vi "Configure Rate.vi"(7 "auto timeout (s)":enum16{"1s", "5s", "10s", "20s"}(ring), 8 "error in":errorcluster, 9 "time (ms)":T1(ring), 10 "option":enum16{"TIME", "AUTO"}(ring), 11 "VISA resource name":refnum<visa-resource-name>) -> (0 "error out":errorcluster, 3 "VISA resource out":refnum<visa-resource-name>)   [LabVIEW 2018, in "Suita SPAW7000.lvlib"]
uses:
  <instrlib>/Suita SPAW7000/Suita SPAW7000.lvlib
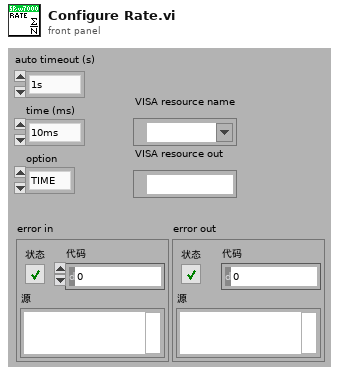
[diagram p1: front panel]
types:
  T1 = enum16{"10ms", "50ms", "100ms", "250ms", "500ms"}
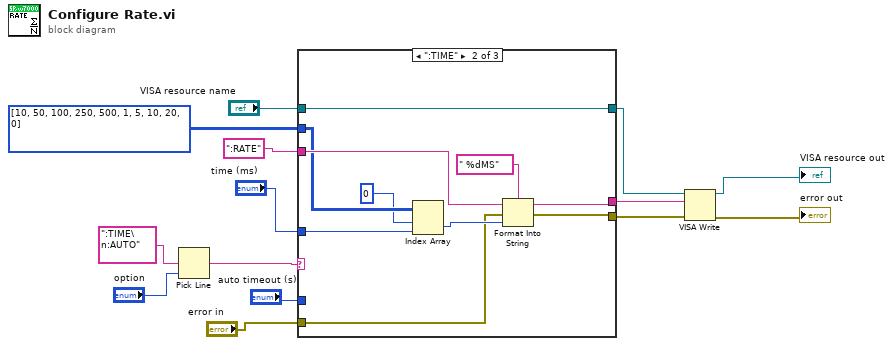
[diagram p0: block diagram]
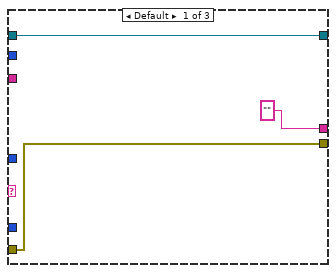
[diagram p2: hidden frame]
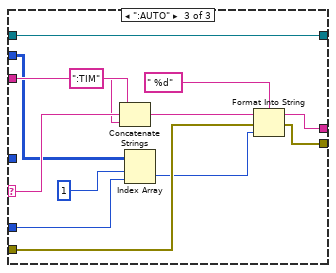
[diagram p3: hidden frame]
diagram:
  n1 = Pick Line(multi-line string=":TIME\n:AUTO", line index="option") -> (output string=w12:string)  [unwired: 1 in]
  n2 = case shown="\":TIME\"" w12 {
    selector: w12 -> [_ _ w39]
    tunnel: ":RATE" -> [_ w27 w40]
    tunnel: "time (ms)" -> [_ w18 _]
    tunnel: i32[][] [[10, 50, 100, 250, 500], [1, 5, 10, 20, 0]] -> [_ w24 w31]
    tunnel: "error in" -> [w17 w23 w35]
    tunnel: [w17 w22 w34] -> w7
    tunnel: "VISA resource name" -> [w16 w21 w32]
    tunnel: [w16 w21 w32] -> w4
    tunnel: ["" ("写入缓冲区") w20 w33] -> w3
    tunnel: "auto timeout (s)" -> [_ _ w28]
    frame Default {
    }
    frame ":TIME" {
      n3 = Index Array(array=w24, index (row)=0 ("索引 (行)"), index (col)=w18) -> (element=w25:i32)
      n4 = Format Into String(format string=" %dMS" ("格式字符串"), initial string=w27, error in=w23, w25) -> (resulting string=w20:string, error out=w22:errorcluster)
    }
    frame ":AUTO" {
      n5 = Concatenate Strings(w40, w39, ":TIM" ("字符串")) -> (w37:string)
      n6 = Index Array(array=w31, index (row)=1 ("索引 (行)"), index (col)=w28) -> (element=w30:i32)
      n7 = Format Into String(format string=" %d" ("格式字符串"), initial string=w37, error in=w35, w30) -> (resulting string=w33:string, error out=w34:errorcluster)
    }
  }
  n8 = VISA Write(VISA resource name=w4, write buffer=w3, error in (no error)=w7) -> (VISA resource name out=→"VISA resource out":refnum<visa-resource-name>, error out=→"error out":errorcluster)  [unwired: 1 out]
